vi "ConfigFIFO.vi"(6 "Used Model Array":T3[](array[typedef]) {"Bus Number" min=-1 max=255 step=1; "Base I/O Addr" format="%.0x"; "Init Status" min=-10 max=0 step=1; "in Use" min=-1 max=1 step=1; "Slot Number" min=-1 max=255 step=1; "Module Type" items=["SPC-600"=600, "SPC-630"=630, "SPC-700"=700, "SPC-730"=730, "SPC-130"=130, "SPC-830"=830, "SPC-140"=140, "SPC-930"=930, "DPC-230"=230, "SPC-150"=150, "SPC-150 N"=151, "SPC-150 NX"=152, "SPC-130 EM"=131, "SPC-130 EMN"=132, "SPC-130IN"=135, "SPC-130INX"=136, "SPC-130INXX"=137, "SPC-160"=160, "SPC-160 X"=161, "SPC-160 PCIE"=162, "SPC-180 N"=180, "SPC-180 NX"=181, "SPC-180 NXX"=182, "SPC-180 N-USB"=185, "SPC-180 NX-USB"=186, "SPC-180 NXX-USB"=187, "SPC-QC-104"=104, "SPC-QC-004"=4, "SPC-QC-106"=106, "DPC-330"=330, "PMS-800"=800, "SPC-590"=590, "Simulation"=-1]}, 7 "User Input":T2={"tac_range"=50.0, "tac_gain"=2, "tac_offset"=0.0, "tac_limit_high"=80.0, "tac_limit_low"=10.0, "collect_time"=2.0, "sync_threshold"=-20.0, "sync_zc_level"=0.0, "sync_freq_div"=4, "cfd_limit_low"=0.0, "cfd_zc_level"=0.0} {"sync_freq_div" items=["1"=1, "2"=2, "4"=4]; "cfd_zc_level" min=-96 max=96 step=0.1 format="%#_3g"; "cfd_limit_low" min=-500 max=0 step=0.1 format="%#_3g"; "sync_zc_level" min=-96 max=96 step=0.1 format="%#_3g"; "sync_threshold" min=-500 max=-20 step=0.1 format="%#_3g"; "tac_limit_low" format="%.3g"; "tac_limit_high" min=0 max=100 step=0.1 format="%.3g"; "collect_time" min=1e-07 max=100000 step=0.001; "tac_offset" min=0 max=100 step=0.1 format="%.4g"; "tac_gain" min=1 max=15 step=1; "tac_range" format="%^#_6g"}, 8 "Error In":errorcluster, 10 "Module No":i16 min=0 max=7 step=1, 11 "DLL Path":path) -> (0 "Error Out":errorcluster, 2 "Module No":i16 min=0 max=7 step=1, 3 "DLL Path":path, 5 "SPC Data":T1={"base_adr"=896, "init"=0, "cfd_limit_low"=5.0, "cfd_limit_high"=80.0, "cfd_zc_level"=0.0, "cfd_holdoff"=5.0, "sync_zc_level"=0.0, "sync_holdoff"=4.0, "sync_threshold"=-20.0, "tac_range"=50.0, "sync_freq_div"=1, "tac_gain"=1, "tac_offset"=0.0, "tac_limit_low"=10.0, "tac_limit_high"=80.0, "adc_resolution"=12, "ext_latch_delay"=0, "collect_time"=0.01, "display_time"=1.0, "repeat_time"=10.0001, "stop_on_time"=1, "stop_on_ovfl"=1, "dither_range"=0, "count_incr"=1, "mem_bank"=0, "dead_time_comp"=1, "scan_control"=61440, "routing_mode"=0, "tac_enable_hold"=10.0, "pci_card_no"=-1, "mode"=0, "scan_size_x"=1, "scan_size_y"=1, "scan_rout_x"=1, "scan_rout_y"=1, "scan_flyback"=0, "scan_borders"=0, "scan_polarity"=0, "pixel_clock"=0, "line_compression"=1, "trigger"=0, "pixel_time"=5e-08, "ext_pixclk_div"=1, "rate_count_time"=1.0, "macro_time_clk"=0, "add_select"=0, "test_eep"=0, "adc_zoom"=0, "img_size_x"=1, "img_size_y"=1, "img_rout_x"=1, "img_rout_y"=1, "xy_gain"=1, "master_clock"=0, "adc_sample_delay"=0, "detector_type"=1, "chan_enable"=4191231, "chan_slope"=0, "chan_spec_no"=34835, "tdc_control"=0, "tdc_offset1"=0.0, "tdc_offset2"=0.0, "tdc_offset3"=0.0, "tdc_offset4"=0.0, "tdc_offset5"=0.0, "tdc_offset6"=0.0, "cfd_th5_tdc"=0.0, "cfd_th6_tdc"=0.0, "cfd_zc5_tdc"=0.0, "cfd_zc6_tdc"=0.0, "future_reserve1"=0, "future_reserve2"=0, "future_reserve3"=0, "future_reserve4"=0} {"chan_spec_no" format="%x"; "chan_enable" format="%x"})   [LabVIEW 2017]
doc: "This VI is a wrapper for the SPC_get_parameters.vi and SPC_set_parameters.vi. \nThe 'User Input' as well as the correct mode code for FIFO operations at the current module type are set for convenience.\nIn FIFO modes 12 is the only correct value for adc_resolution in SPCData.\nYou might want to try different values for dither_range.\nstop_on_time and stop_on_ovl might need different values in your setup.\n\ninfo@becker-hickl.com"
uses:
  SPC_Controls/SPCModInfo.ctl
  SPC_Controls/ModuleType.ctl
  Examples/Example_Controls/UserInput.ctl
  SPC_Controls/SPCdata.ctl
  SPC_Controls/dither_range.ctl
  SPC_Controls/macro_time_clk.ctl
panel:
  # "TAC / Time Range"
  # "CFD"
  # "(start)"
  # "SYNC"
  # "(stop)"
  # "range"
  # "gain"
  # "threshold(LL)"
  # "offset"
  # "limit high"
  # "limit low"
  # "zero cross(ZC)"
  # "Collection Time"
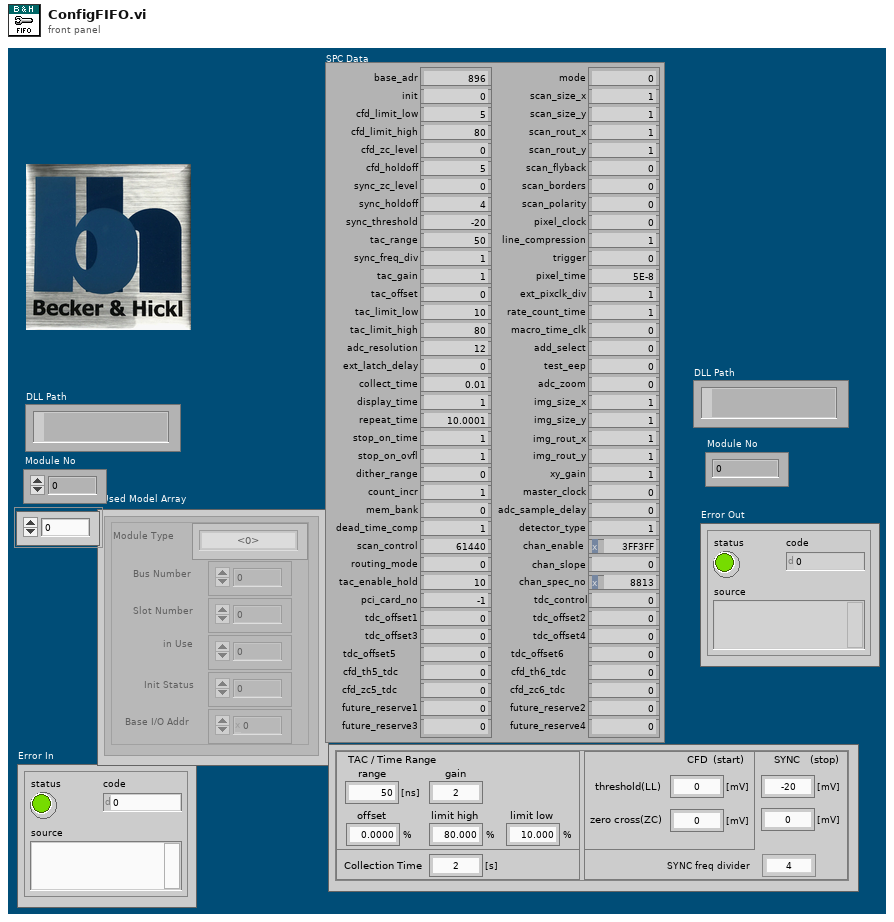
[diagram p1: front panel]
types:
  T1 = typedef "SPCdata.ctl" = cluster{"base_adr":u16, "init":i16, "cfd_limit_low":sgl, "cfd_limit_high":sgl, "cfd_zc_level":sgl, "cfd_holdoff":sgl, "sync_zc_level":sgl, "sync_holdoff":sgl, "sync_threshold":sgl, "tac_range":sgl, "sync_freq_div":i16, "tac_gain":i16, "tac_offset":sgl, "tac_limit_low":sgl, "tac_limit_high":sgl, "adc_resolution":i16, "ext_latch_delay":i16, "collect_time":sgl, "display_time":sgl, "repeat_time":sgl, "stop_on_time":i16, "stop_on_ovfl":i16, "dither_range":i16, "count_incr":i16, "mem_bank":i16, "dead_time_comp":i16, "scan_control":u16, "routing_mode":u16, "tac_enable_hold":sgl, "pci_card_no":i16, "mode":u16, "scan_size_x":u32, "scan_size_y":u32, "scan_rout_x":u32, "scan_rout_y":u32, "scan_flyback":u32, "scan_borders":u32, "scan_polarity":u16, "pixel_clock":u16, "line_compression":u16, "trigger":u16, "pixel_time":sgl, "ext_pixclk_div":u32, "rate_count_time":sgl, "macro_time_clk":i16, "add_select":i16, "test_eep":i16, "adc_zoom":i16, "img_size_x":u32, "img_size_y":u32, "img_rout_x":u32, "img_rout_y":u32, "xy_gain":i16, "master_clock":i16, "adc_sample_delay":i16, "detector_type":i16, "chan_enable":u32, "chan_slope":u32, "chan_spec_no":u32, "tdc_control":u32, "tdc_offset1":sgl, "tdc_offset2":sgl, "tdc_offset3":sgl, "tdc_offset4":sgl, "tdc_offset5":sgl, "tdc_offset6":sgl, "cfd_th5_tdc":sgl, "cfd_th6_tdc":sgl, "cfd_zc5_tdc":sgl, "cfd_zc6_tdc":sgl, "future_reserve1":u64, "future_reserve2":u64, "future_reserve3":u64, "future_reserve4":u64}
  T2 = typedef "UserInput.ctl" = cluster{"tac_range":sgl, "tac_gain":i16, "tac_offset":sgl, "tac_limit_high":sgl, "tac_limit_low":sgl, "collect_time":sgl, "sync_threshold":sgl, "sync_zc_level":sgl, "sync_freq_div":i16, "cfd_limit_low":sgl, "cfd_zc_level":sgl}
  T3 = typedef "SPCModInfo.ctl" = cluster{"Module Type":T4, "Bus Number":i16, "Slot Number":i16, "in Use":i16, "Init Status":i16, "Base I/O Addr":u16}
  T4 = typedef "ModuleType.ctl" = i16
  T5 = typedef "macro_time_clk.ctl" = enum16{"25ns", "Sync", "1/2 Sync", "1/4 Sync", "1/8 Sync"}
  T6 = typedef "dither_range.ctl" = i16
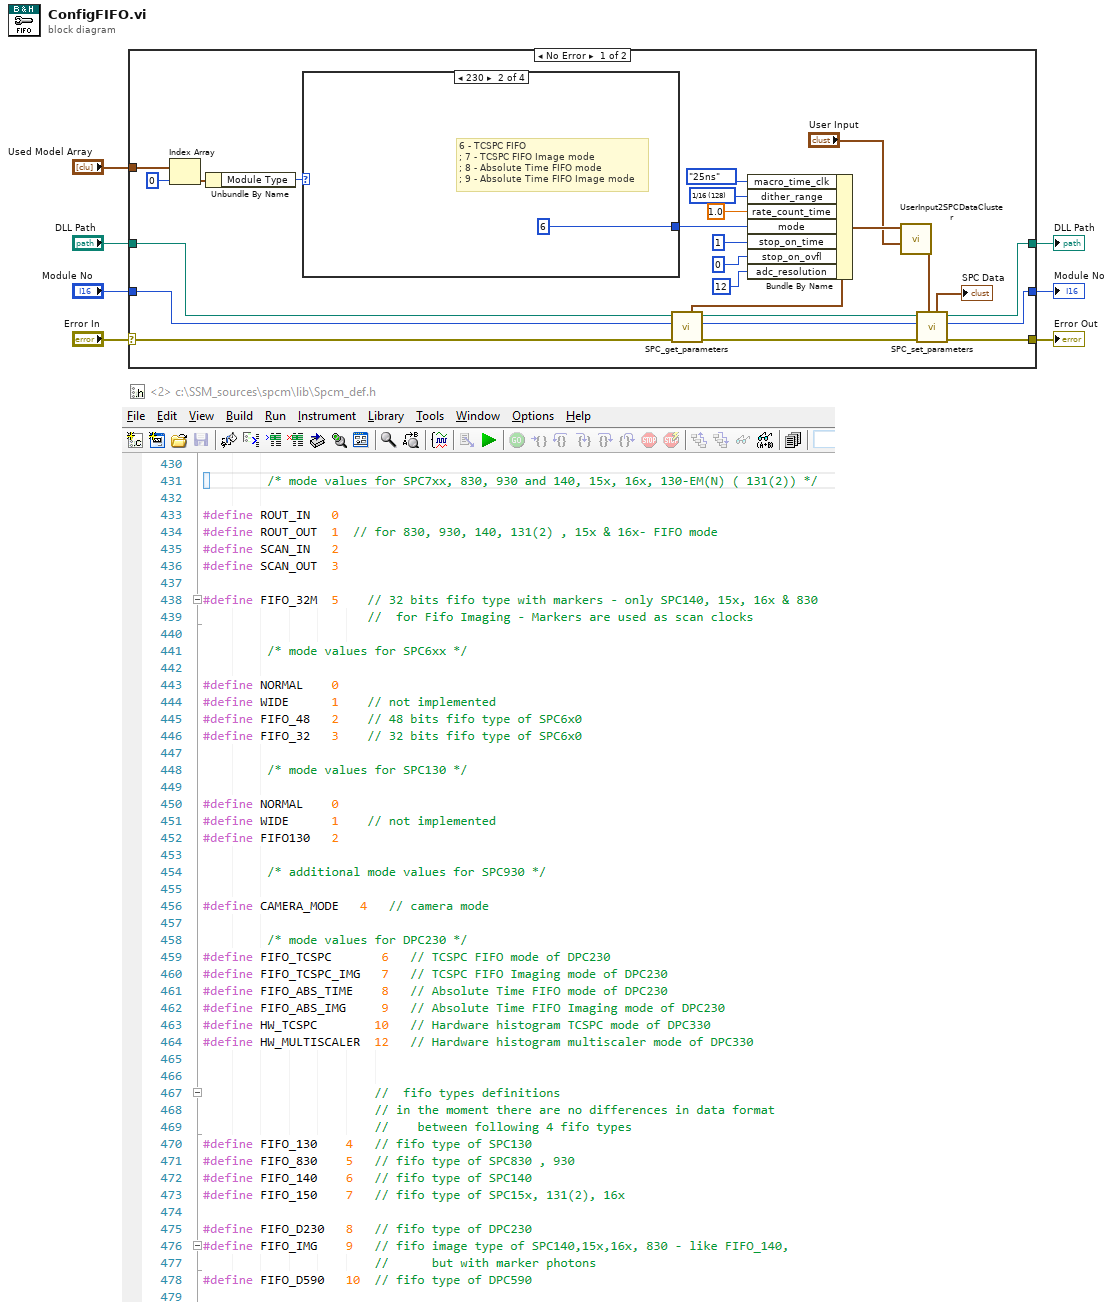
[diagram p0: block diagram]
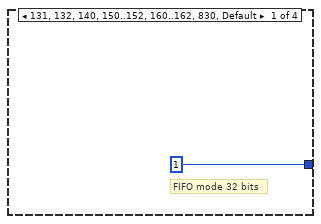
[diagram p2: hidden frame]
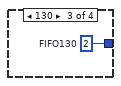
[diagram p3: hidden frame]
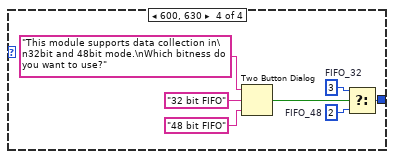
[diagram p4: hidden frame]
diagram:
  n1 = case shown="No Error" "Error In" {
    selector: "Error In" -> [w28 w45]
    tunnel: [w27 w43] -> w6
    tunnel: "DLL Path" -> [w26 w43]
    tunnel: "Module No" -> [w25 w44]
    tunnel: [w24 w44] -> w3
    tunnel: [w23 w45] -> w2
    tunnel: "Used Model Array" -> [w11 _]
    frame No Error {
      w9 = T6 128 items=["0"=0, "1/64"=32, "1/32"=64, "1/16"=128, "1/8"=256] ("DithRange")
      n2 = Index Array(array=w11, index=0) -> (element=w18:T3)
      n3 = Unbundle By Name(w18) -> ("Module Type"=w20:T4)
      n4 = case shown="230" w20 {
        tunnel: [u16 1 ("Parameter Value") u16 6 ("Parameter Value") w35 w37] -> w30
        frame 131, 132, 140, 150..152, 160..162, 830, Default {
          # "FIFO mode 32 bits"
        }
        frame 230 {
          # "6 - TCSPC FIFO\n; 7 - TCSPC FIFO Image mode\n; 8 - Absolute Time FIFO mode\n; 9 - Absolute Time FIFO Image mode"
        }
        frame 130 {
          w35 = u16 2  # FIFO130
        }
        frame 600, 630 {
          w38 = u16 3  # FIFO_32
          w39 = u16 2  # FIFO_48
          n5 = Two Button Dialog(message="This module supports data collection in\n32bit and 48bit mode.\nWhich bitness do you want to use?", 1:"48 bit FIFO" ("T button name (\"OK\")"), 2:"32 bit FIFO" ("T button name (\"OK\")")) -> (T button?=w36:bool)
          n6 = Select(t=w38, s=w36, f=w39) -> (s? t:f=w37:u16)
        }
      }
      n7 = call "SPC_get_parameters.vi"("Error In"=w28, "Module No"=w25, "DLL Path"=w26) -> ("Error Out"=w12:errorcluster, "Module No"=w13:i16, "DLL Path"=w14:path, "SPCdata"=w29:T1)  [unwired: 5 in]
      n8 = Bundle By Name(cluster=w29, "macro_time_clk"=macro_time_clk."25ns", "dither_range"=w9, "rate_count_time"=sgl 1.0, "mode"=w30, "stop_on_time"=i16 1 ("Stop on Time"), "stop_on_ovfl"=i16 0 ("Stop on Overflow"), "adc_resolution"=i16 12 ("ADC Resolution")) -> (w16:T1)
      n9 = call "UserInput2SPCDataCluster.vi"("UserInput_In"="User Input", "SPCData_In"=w16) -> ("SPCData_Out"=w17:T1)  [unwired: 9 in]
      n10 = call "SPC_set_parameters.vi"("SPCdata In"=w17, "Error In"=w12, "Module No."=w13, "DLL Path"=w14) -> ("Error Out"=w23:errorcluster, "Module No"=w24:i16, "DLL Path"=w27:path, "SPCdata Out"=→"SPC Data":T1)  [unwired: 4 in]
    }
    frame Error {
    }
  }
  "Error Out" <- w2
  "DLL Path" <- w6
  "Module No" <- w3
